vi "diffImages.vi"(8 "error in (no error)":errorcluster, 10 "Image 2":T1, 11 "Image 1":T1) -> (0 "error out":errorcluster, 2 "Images Same?":bool, 3 "Diff Image Data":T1)   [LabVIEW 2018, in "Image_Diff.lvlib"]
doc: "This VI subtracts Image 2 from Image 1 and searches for differences. If there are any, it paints them red and outputs a FALSE on ImagesSame?"
uses:
  Image_Diff.lvlib
  <vilib>/picture/picture.llb/imagedata.ctl
panel:
  out "Diff Image":picture
  out "Image 2":picture
  out "Image 1":picture
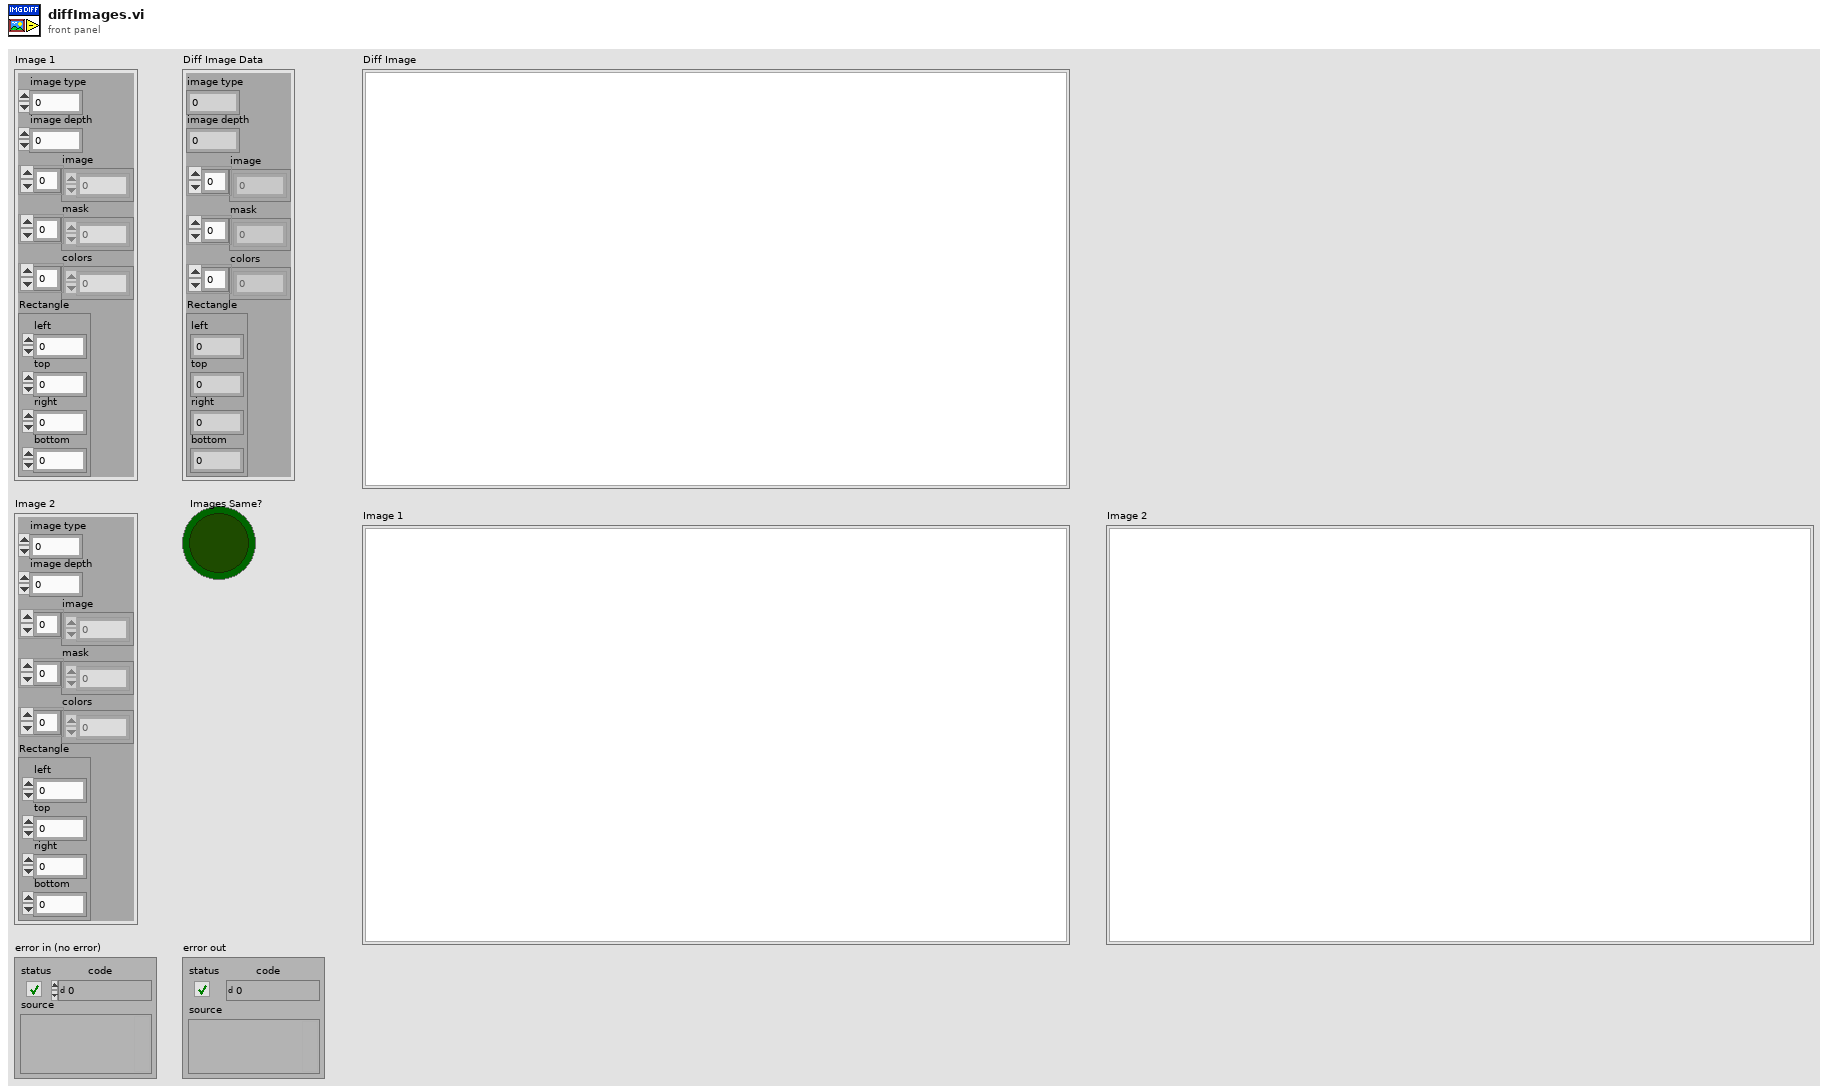
[diagram p1: front panel]
types:
  T1 = typedef "imagedata.ctl" = cluster{"image type":i32, "image depth":i32, "image":u8[], "mask":u8[], "colors":u32[], "Rectangle":cluster{"left":i16, "top":i16, "right":i16, "bottom":i16}}
  T2 = enum32{"Invalid", "Standard", "Closed", "Hidden", "Minimized", "Maximized"}
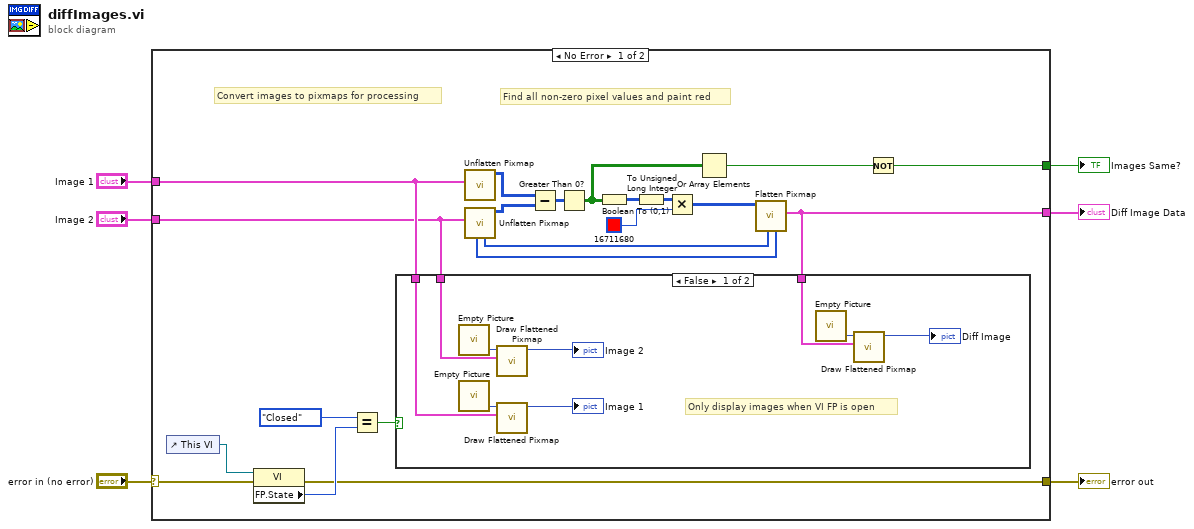
[diagram p0: block diagram]
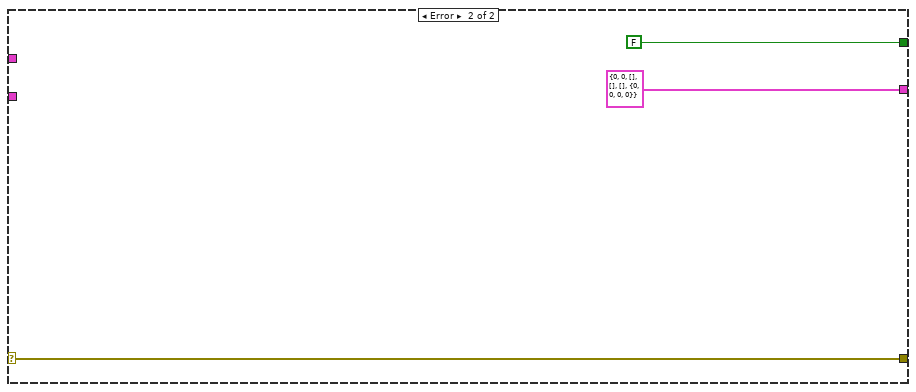
[diagram p3: hidden frame]
diagram:
  n1 = case shown="No Error" "error in (no error)" {
    selector: "error in (no error)" -> [w18 w39]
    tunnel: [w7 FALSE] -> w6
    tunnel: "Image 1" -> [w20 _]
    tunnel: "Image 2" -> [w19 _]
    tunnel: [w17 w39] -> w2
    tunnel: [w10 T1 {"image type"=0, "image depth"=0, "image"=[], "mask"=[], "colors"=[], "Rectangle"={"left"=0, "top"=0, "right"=0, "bottom"=0}} ("image data")] -> w1
    frame No Error {
      # "Find all non-zero pixel values and paint red"
      # "Convert images to pixmaps for processing"
      n2 = control-ref of="This VI"() -> (w24:refnum<vi>)
      n3 = property class="VI"(reference=w24, error in=w18) -> (error out=w17:errorcluster, "FP.State"=w23:T2)  [unwired: 1 out]
      n4 = Equal?(x=T2."Closed" ("y"), y=w23) -> (x = y?=w21:bool)
      n5 = call <vilib>:"Unflatten Pixmap.vi"("image data"=w20) -> ("24-bit pixmap"=w9:u32[][])  [unwired: 4 in, 6 out]
      n6 = call <vilib>:"Unflatten Pixmap.vi"("image data"=w19) -> ("24-bit pixmap"=w8:u32[][], "colors"=w14:u32[], "mask"=w13:u8[])  [unwired: 4 in, 4 out]
      n7 = Subtract(x=w9, y=w8) -> (x-y=w27:u32[][])
      n8 = Greater Than 0?(x=w27) -> (x > 0?=w12:bool[][])
      n9 = Boolean To (0,1)(Boolean=w12) -> (0, 1=w26:i16[][])
      n10 = To Unsigned Long Integer(number=w26) -> (unsigned 32bit integer=w16:u32[][])
      n11 = Multiply(x=w16, y=u32 16711680) -> (x*y=w15:u32[][])
      n12 = Or Array Elements(Boolean array=w12) -> (logical OR=w11:bool)
      n13 = call <vilib>:"Flatten Pixmap.vi"("mask"=w13, "colors"=w14, "24-bit pixmap"=w15) -> ("image data"=w10:T1)  [unwired: 8 in]
      n14 = case shown="False" w21 {
        tunnel: w20 -> [w32 _]
        tunnel: w19 -> [w31 _]
        tunnel: w10 -> [w28 _]
        frame False {
          # "Only display images when VI FP is open"
          n15 = call "Empty Picture"() -> ("empty picture"=w33:picture)
          n16 = call "Empty Picture"() -> ("empty picture"=w34:picture)
          n17 = call <vilib>:"Draw Flattened Pixmap.vi"("image data"=w31, "picture"=w33) -> ("new picture"=→"Image 2":picture)  [unwired: 7 in]
          n18 = call <vilib>:"Draw Flattened Pixmap.vi"("image data"=w32, "picture"=w34) -> ("new picture"=→"Image 1":picture)  [unwired: 7 in]
          n19 = call "Empty Picture"() -> ("empty picture"=w30:picture)
          n20 = call <vilib>:"Draw Flattened Pixmap.vi"("image data"=w28, "picture"=w30) -> ("new picture"=→"Diff Image":picture)  [unwired: 7 in]
        }
        frame True {
        }
      }
      n21 = Not(x=w11) -> (.not. x?=w7:bool)
    }
    frame Error {
    }
  }
  "Images Same?" <- w6
  "error out" <- w2
  "Diff Image Data" <- w1
